vi "Stamping Motion.vi"(7 "Console Log in":refnum<class "Console Log.lvclass">, 8 "error in":errorcluster, 11 "Gluing Procedure in":refnum<class "Gluing Procedure.lvclass">) -> (0 "error out":errorcluster, 1 "Step canceled?":bool, 3 "Gluing Procedure out":refnum<class "Gluing Procedure.lvclass">, 5 "Console Log out":refnum<class "Console Log.lvclass">)   [LabVIEW 2017, in "Gluing Procedure.lvclass"]
uses:
  Gluing Procedure.lvclass
  Type Definitions/Stamping.ctl
  Shared Components/GrabberTool Class/GrabberTool Class.lvclass
  Application Utilities/Console Log/Console Log.lvclass
panel:
  # "This VI does the stamping motion\n1.  grab stamp\n2. dip stamp\n3. apply stamp\n4. return stamp\n\nPulls Stamp -> Glue -> BBM path motion (chuck/slot)"
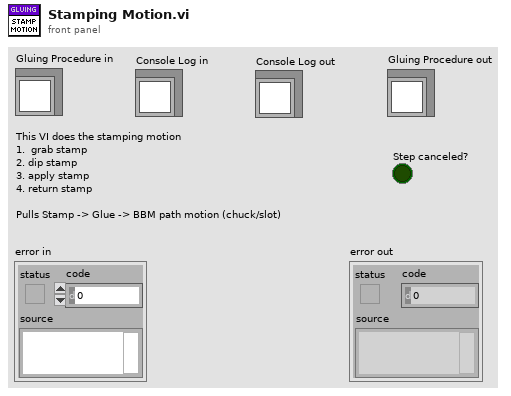
[diagram p1: front panel]
types:
  T1 = typedef "Stamping.ctl" = cluster{"Has been run?":bool}
  T2 = typedef "Configure.ctl" = cluster{"Has been run?":bool, "Active Paths":T3, "Glue Pathways":T4, "Chuck Module Used for BBM:":T6}
  T3 = typedef "Active Paths.ctl" = bool[]
  T4 = typedef "Glue Paths.ctl" = T5[]
  T5 = typedef "Glue Path.ctl" = cluster{"HDI Slot ":i32, "Stamp Slot":i32, "Glue Slot":i32, "Weight Slot":i32, "BBM Slot":i32}
  T6 = typedef "BBM Chuck Used.ctl" = i32
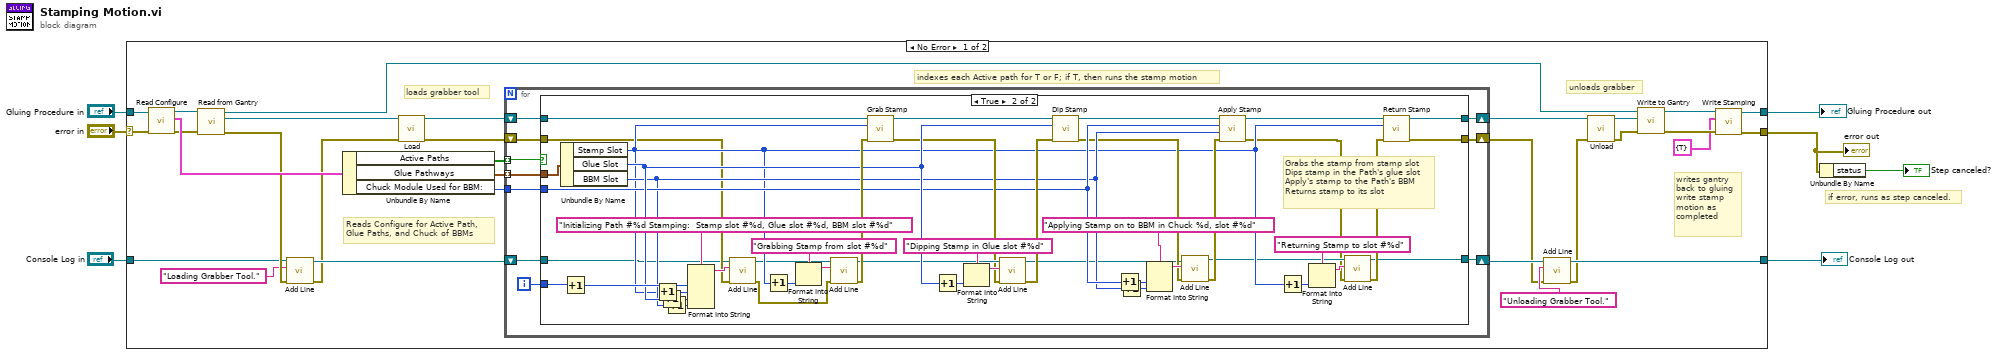
[diagram p0: block diagram]
diagram:
  # "if error, runs as step canceled."
  n1 = case shown="No Error" "error in" {
    selector: "error in" -> [w35 w99]
    tunnel: [w18 w99] -> w2
    tunnel: [w37 w98] -> w5
    tunnel: "Gluing Procedure in" -> [w36 w98]
    tunnel: "Console Log in" -> [w14 w97]
    tunnel: [w11 w97] -> w3
    frame No Error {
      # "indexes each Active path for T or F; if T, then runs the stamp motion"
      # "writes gantry\nback to gluing\nwrite stamp \nmotion as \ncompleted"
      # "unloads grabber"
      # "loads grabber tool"
      # "Reads Configure for Active Path, \nGlue Paths, and Chuck of BBMs"
      n2 = call "Read Configure.vi"("error in (no error)"=w35, "Gluing Procedure in"=w36) -> ("error out"=w29:errorcluster, "Configure"=w34:T2, "Gluing Procedure out"=w31:refnum<class "Gluing Procedure.lvclass">)  [unwired: 7 in]
      n3 = call "Read from Gantry.vi"("error in (no error)"=w29, "Gluing Procedure in"=w31) -> ("error out"=w15:errorcluster, "Gantry"=w30:refnum<class "Gantry Class.lvclass">, "Gluing Procedure out"=w23:refnum<class "Gluing Procedure.lvclass">)  [unwired: 7 in]
      n4 = call "Add Line.vi"("error in"=w15, "String"="Loading Grabber Tool.", "Console Log in"=w14) -> ("error out"=w16:errorcluster, "Console Log out"=w17:refnum<class "Console Log.lvclass">)  [unwired: 7 in]
      n5 = Unbundle By Name(w34) -> ("Active Paths"=w33:T3, "Glue Pathways"=w32:T4, "Chuck Module Used for BBM:"=w26:T6)
      n6 = call "Load.vi"("error in"=w16, "Gantry In"=w30) -> ("error out"=w27:errorcluster, "Grabber Tool out"=w28:refnum<class "GrabberTool Class.lvclass">)  [unwired: 8 in]
      n7 = for {
        tunnel: w33 -> [w47] mode=indexing
        tunnel: w32 -> [w46] mode=indexing
        shift-right: [w43] -> w25
        shift-left: w28 -> [w44]
        shift-right: [w42] -> w9
        shift-left: w27 -> [w45]
        tunnel: w26 -> [w41]
        shift-right: [w38] -> w12
        shift-left: w17 -> [w39]
        i -> [w40]
        n8 = case shown="True" w47 {
          tunnel: w46 -> [_ w90]
          tunnel: w45 -> [w49 w54]
          tunnel: w44 -> [w50 w96]
          tunnel: [w50 w92] -> w43
          tunnel: [w49 w91] -> w42
          tunnel: w41 -> [_ w69]
          tunnel: w40 -> [_ w89]
          tunnel: w39 -> [w48 w53]
          tunnel: [w48 w56] -> w38
          frame False {
          }
          frame True {
            # "Grabs the stamp from stamp slot\nDips stamp in the Path's glue slot\nApply's stamp to the Path's BBM\nReturns stamp to its slot"
            n9 = Unbundle By Name(w90) -> ("Stamp Slot"=w60:i32, "Glue Slot"=w79:i32, "BBM Slot"=w67:i32)
            n10 = Increment(x=w89) -> (x+1=w88:i32)
            n11 = Increment(x=w60) -> (x+1=w85:i32)
            n12 = Increment(x=w79) -> (x+1=w84:i32)
            n13 = Increment(x=w67) -> (x+1=w83:i32)
            n14 = Format Into String(format string="Initializing Path #%d Stamping:  Stamp slot #%d, Glue slot #%d, BBM slot #%d", w88, w85, w84, w83) -> (resulting string=w55:string)  [unwired: 2 in, 1 out]
            n15 = call "Add Line.vi"("error in"=w54, "String"=w55, "Console Log in"=w53) -> ("error out"=w51:errorcluster, "Console Log out"=w52:refnum<class "Console Log.lvclass">)  [unwired: 7 in]
            n16 = Increment(x=w60) -> (x+1=w82:i32)
            n17 = Format Into String(format string="Grabbing Stamp from slot #%d", w82) -> (resulting string=w86:string)  [unwired: 2 in, 1 out]
            n18 = call "Add Line.vi"("error in"=w51, "String"=w86, "Console Log in"=w52) -> ("error out"=w80:errorcluster, "Console Log out"=w76:refnum<class "Console Log.lvclass">)  [unwired: 7 in]
            n19 = call "Grab Stamp.vi"("error in"=w80, "Stamp Number"=w60, "GrabberTool in"=w96) -> ("error out"=w74:errorcluster, "GrabberTool out"=w95:refnum<class "GrabberTool Class.lvclass">)  [unwired: 7 in]
            n20 = Increment(x=w79) -> (x+1=w78:i32)
            n21 = Format Into String(format string="Dipping Stamp in Glue slot #%d", w78) -> (resulting string=w75:string)  [unwired: 2 in, 1 out]
            n22 = call "Add Line.vi"("error in"=w74, "String"=w75, "Console Log in"=w76) -> ("error out"=w73:errorcluster, "Console Log out"=w65:refnum<class "Console Log.lvclass">)  [unwired: 7 in]
            n23 = call "Dip Stamp.vi"("error in"=w73, "Reservoir Number"=w79, "GrabberTool in"=w95) -> ("error out"=w66:errorcluster, "GrabberTool out"=w94:refnum<class "GrabberTool Class.lvclass">)  [unwired: 7 in]
            n24 = Increment(x=w69) -> (x+1=w70:T6)
            n25 = Increment(x=w67) -> (x+1=w68:i32)
            n26 = Format Into String(format string="Applying Stamp on to BBM in Chuck %d, slot #%d", w70, w68) -> (resulting string=w72:string)  [unwired: 2 in, 1 out]
            n27 = call "Add Line.vi"("error in"=w66, "String"=w72, "Console Log in"=w65) -> ("error out"=w64:errorcluster, "Console Log out"=w59:refnum<class "Console Log.lvclass">)  [unwired: 7 in]
            n28 = call "Apply Stamp.vi"("error in"=w64, "Slot Number"=w67, "Chuck Number"=w69, "GrabberTool in"=w94) -> ("error out"=w58:errorcluster, "GrabberTool out"=w93:refnum<class "GrabberTool Class.lvclass">)  [unwired: 6 in]
            n29 = Increment(x=w60) -> (x+1=w62:i32)
            n30 = Format Into String(format string="Returning Stamp to slot #%d", w62) -> (resulting string=w61:string)  [unwired: 2 in, 1 out]
            n31 = call "Add Line.vi"("error in"=w58, "String"=w61, "Console Log in"=w59) -> ("error out"=w57:errorcluster, "Console Log out"=w56:refnum<class "Console Log.lvclass">)  [unwired: 7 in]
            n32 = call "Return Stamp.vi"("error in"=w57, "Slot Number"=w60, "GrabberTool in"=w93) -> ("error out"=w91:errorcluster, "GrabberTool out"=w92:refnum<class "GrabberTool Class.lvclass">)  [unwired: 7 in]
          }
        }
      }
      n33 = call "Add Line.vi"("error in"=w9, "String"="Unloading Grabber Tool.", "Console Log in"=w12) -> ("error out"=w8:errorcluster, "Console Log out"=w11:refnum<class "Console Log.lvclass">)  [unwired: 7 in]
      n34 = call "Unload.vi"("error in"=w8, "GrabberTool in"=w25) -> ("error out"=w22:errorcluster, "Gantry out"=w24:refnum<class "Gantry Class.lvclass">)  [unwired: 8 in]
      n35 = call "Write to Gantry.vi"("error in (no error)"=w22, "Gantry"=w24, "Gluing Procedure in"=w23) -> ("error out"=w20:errorcluster, "Gluing Procedure out"=w21:refnum<class "Gluing Procedure.lvclass">)  [unwired: 7 in]
      n36 = call "Write Stamping.vi"("error in (no error)"=w20, "Stamping"=T1 {"Has been run?"=TRUE}, "Gluing Procedure in"=w21) -> ("error out"=w18:errorcluster, "Gluing Procedure out"=w37:refnum<class "Gluing Procedure.lvclass">)  [unwired: 7 in]
    }
    frame Error {
    }
  }
  "error out" <- w2
  "Gluing Procedure out" <- w5
  "Console Log out" <- w3
  n37 = Unbundle By Name(w2) -> ("status"=→"Step canceled?":bool)
